vi "Send Update Sequence Params.vi"(7 "Priority":T3=enum."Normal" caption="Message Priority (Normal)", 8 "error in (no error)":errorcluster, 9 "Daq Channel Info In":T1, 10 "Sequence Parameters In":T2, 11 "Message Enqueuer in":refnum<class "Message Enqueuer.lvclass">) -> (0 "error out":errorcluster, 3 "Message Enqueuer out":refnum<class "Message Enqueuer.lvclass">)   [LabVIEW 2015, in "UI.lvlib" / "Update Sequence Params Msg.lvclass"]
doc: "Sends the <b>UI.lvlib:Update Sequence Params Msg.lvclass</b> message.\n\nThis message will call <b>Update Sequence Params.vi</b> on the <b>UI.lvlib:UI.lvclass</b> actor.\n\n<b>Update Sequence Params.vi Description</b>"
uses:
  Update Sequence Params Msg.lvclass
  <vilib>/ActorFramework/Message Enqueuer/Message Enqueuer.lvclass
  <vilib>/ActorFramework/Message Enqueuer/Message Priority.ctl
  Sequencer/Sequencer/Sequence Parameters.ctl
  Sequencer/Sequencer/Daq Channel Info.ctl
  Update Sequence Params Msg.lvclass/Update Sequence Params Msg.ctl
  <vilib>/ActorFramework/Message Enqueuer/Message Enqueuer.lvclass/Message Enqueuer.ctl
  <vilib>/ActorFramework/Message Priority Queue/Priority Enqueue.vi
  Sequencer/Sequencer/Sequencer.lvclass
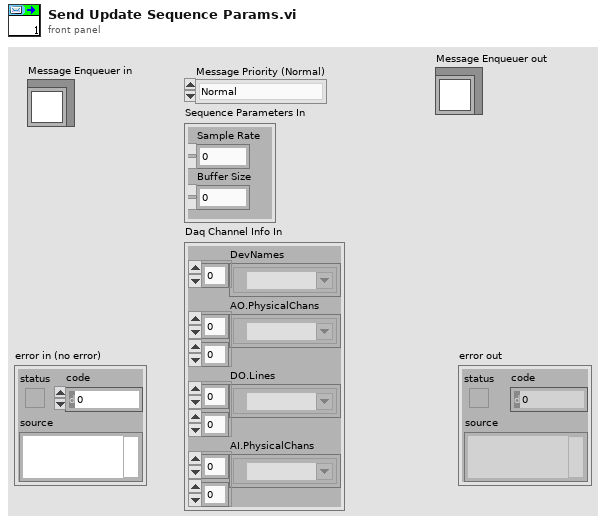
[diagram p1: front panel]
types:
  T1 = typedef "Sequencer.lvlib/Sequencer.lvclass/Daq Channel Info.ctl" = cluster{"DevNames":tag[], "AO.PhysicalChans":tag[][], "DO.Lines":tag[][], "AI.PhysicalChans":tag[][]}
  T2 = typedef "Sequencer.lvlib/Sequencer.lvclass/Sequence Parameters.ctl" = cluster{"Buffer Size":dbl, "Sample Rate":dbl}
  T3 = typedef "Actor Framework.lvlib/Message Enqueuer.lvclass/Message Priority.ctl" = enum16{"Low", "Normal", "High"}
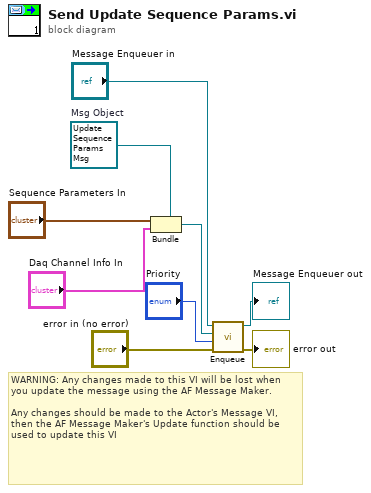
[diagram p0: block diagram]
diagram:
  w7 = refnum<class "Update Sequence Params Msg.lvclass"> refnum  # Msg Object
  # "WARNING: Any changes made to this VI will be lost when you update the message using the AF Message Maker.\n\nAny changes should be made to the Actor's Message VI, then the AF Message Maker's Update function should be used to update this VI"
  n1 = Bundle(cluster=w7, "Sequence Parameters In", "Daq Channel Info In") -> (w2:refnum<class "Update Sequence Params Msg.lvclass">)
  n2 = call <vilib>:"Enqueue.vi"("error in (no error)"="error in (no error)", "Message Priority (Normal)"="Priority", "Message"=w2, "Message Enqueuer in"="Message Enqueuer in") -> ("error out"=→"error out":errorcluster, "Message Enqueuer out"=→"Message Enqueuer out":refnum<class "Message Enqueuer.lvclass">)  [unwired: 6 in]
